vi "Host3.vi"() -> ()   [LabVIEW 2025]
uses:
  <vilib>/numeric/Random Number (Range) U64.vi
  <vilib>/Analysis/baseanly.llb/Real Dot Product.vi
  <vilib>/Analysis/baseanly.llb/Real A x B.vi
  <vilib>/numeric/sub_Random U32.vi
  <vilib>/Analysis/Matrix/Numeric/Conversions/Matrix To Array - RM.vi
  <vilib>/FPGAPlugInAG/cRIO-9033/niLvFpga_Open_cRIO-9033.vi
  <vilib>/rvi/interface/common/dynamic/niFpgaDynamicAddResources.vi
  <vilib>/FPGAPlugInAG/Dynamic/niLvFpga_Reset_Dynamic.vi
  <vilib>/Utility/error.llb/Error Cluster From Error Code.vi
  <vilib>/rvi/errors/niLvFpgaAdjustHostInterfaceError.vi
  <vilib>/FPGAPlugInAG/Dynamic/niLvFpga_Run_Dynamic.vi
  <vilib>/FPGAPlugInAG/Dynamic/niLvFpga_Close_Dynamic.vi
  <vilib>/rvi/interface/nirviOpenFPGA/nirviOpenFPGA.xnode
  FPGA Bitfiles/dotplot9033_FPGATarget_Target2_D+o9JZmHLrs.lvbitx
  Target2.vi
  <vilib>/rvi/interface/nirviMethod/nirviMethod.xnode
  <vilib>/rvi/interface/nirviReadWriteControl/nirviReadWriteControl.xnode
  <vilib>/rvi/interface/nirviCloseFPGA/nirviCloseFPGA.xnode
  <vilib>/rvi/errors/niLvFpgaMergeErrorWithErrorCode.vi
  <vilib>/Analysis/NI_AALBase.lvlib
  <vilib>/Analysis/Matrix/NI_Matrix.lvlib
  <vilib>/FPGAPlugInAG/Dynamic/niLvFpga_WriteFifo_Dynamic.vi
  <vilib>/FPGAPlugInAG/Dynamic/niLvFpga_ReadFifo_Dynamic.vi
  NiFpgaLv.dll
  <vilib>/rvi/interface/Simulation/niFpgaSimulationCallBeginRW.vi
panel:
  out "FIFO D.2 Output":fxp<+/-,32,16>[](array[numeric])
  out "Elements Remaining 4":u32
  out "FIFO C.2 Output":fxp<+/-,32,16>[](array[numeric])
  out "Elements Remaining 3":u32
  out "FIFO D Output":fxp<+/-,32,16>[](array[numeric])
  out "Elements Remaining 2":u32
  out "Array 1.2":fxp<+/-,32,16>[](array[numeric])
  out "Array 2.1":fxp<+/-,32,16>[](array[numeric])
  out "Array 2":fxp<+/-,32,16>[](array[numeric])
  out "Array 1":fxp<+/-,32,16>[](array[numeric])
  out "element 4":fxp<+/-,32,16>
  out "element 3":fxp<+/-,32,16>
  out "element 2":fxp<+/-,32,16>
  out "element":fxp<+/-,32,16>
  out "interleaved array 2":fxp<+/-,32,16>[](array[numeric])
  out "interleaved array":fxp<+/-,32,16>[](array[numeric])
  out "Case Number":i16
  out "Numeric":i32
  out "appended array 2":fxp<+/-,32,16>[](array[numeric])
  out "appended array":fxp<+/-,32,16>[](array[numeric])
  out "cr":fxp<+/-,32,16>[](array[numeric])
  out "Elements Remaining":u32
  out "FIFO C Output":fxp<+/-,32,16>[](array[numeric])
  out "FIFO A Input":fxp<+/-,32,16>[](array[numeric])
  out "FIFO B Input":fxp<+/-,32,16>[](array[numeric])
  out "X * Y":fxp<+/-,64,32>
  out "elements in B":i32
  out "elements in A":i32
  out "sum of error":dbl
  out "C - FPGA code":fxp<+/-,32,16>[][](array[numeric])
  out "elements in C":i32
  out "C - Real":dbl[][](array[numeric])
  out "B":fxp<+/-,32,16>[][](array[numeric])
  out "A":fxp<+/-,32,16>[][](array[numeric])
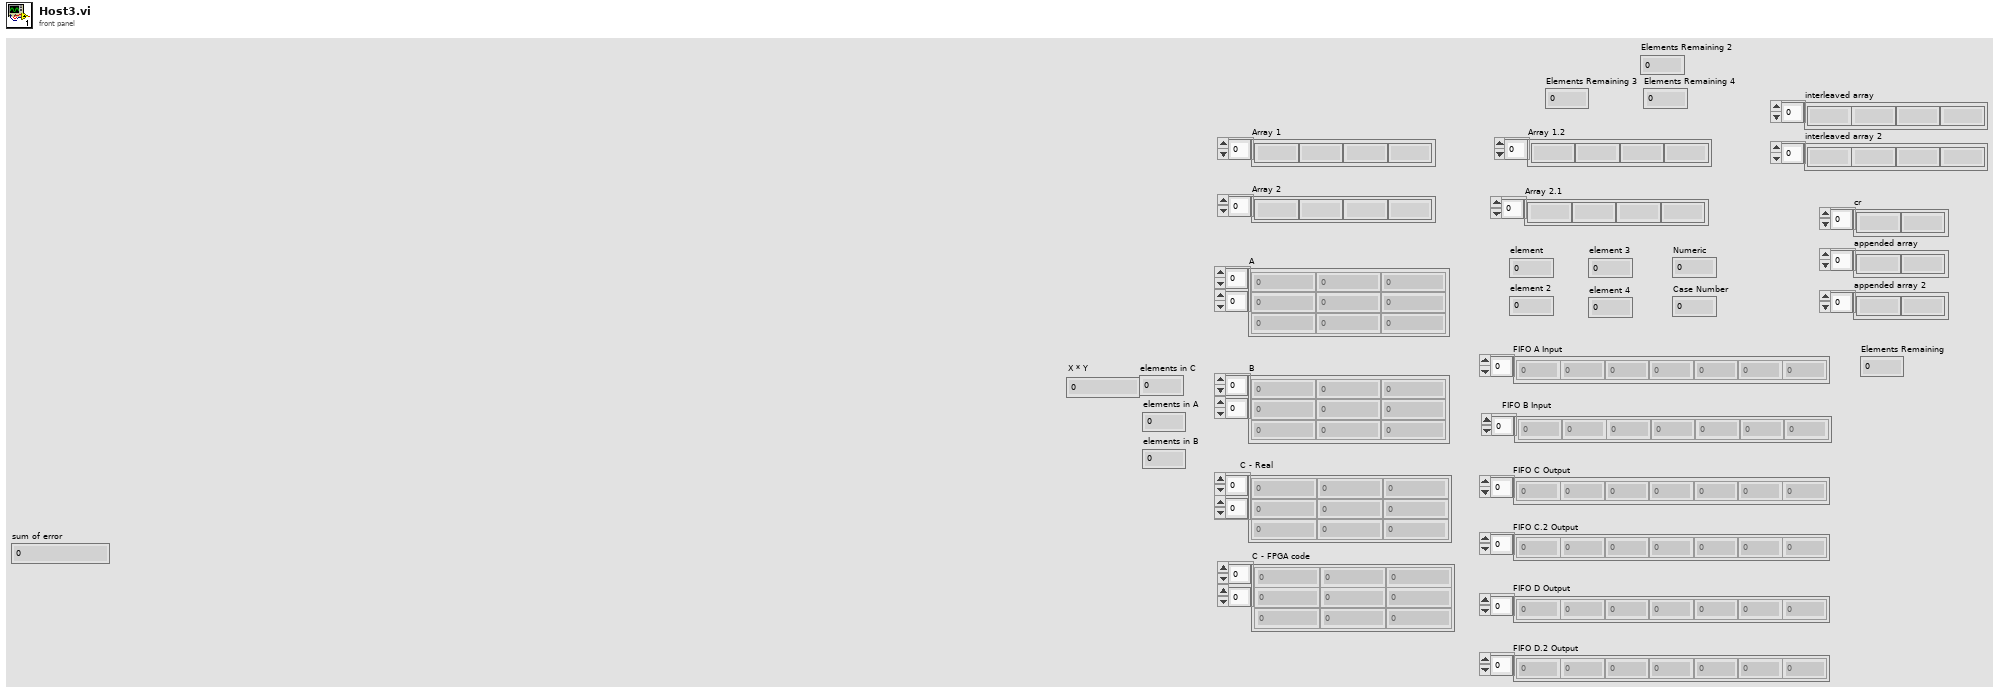
[diagram p1: front panel]
types:
  T1 = typedef "NI_Matrix.lvlib/RealMatrix.ctl" = dbl[][]
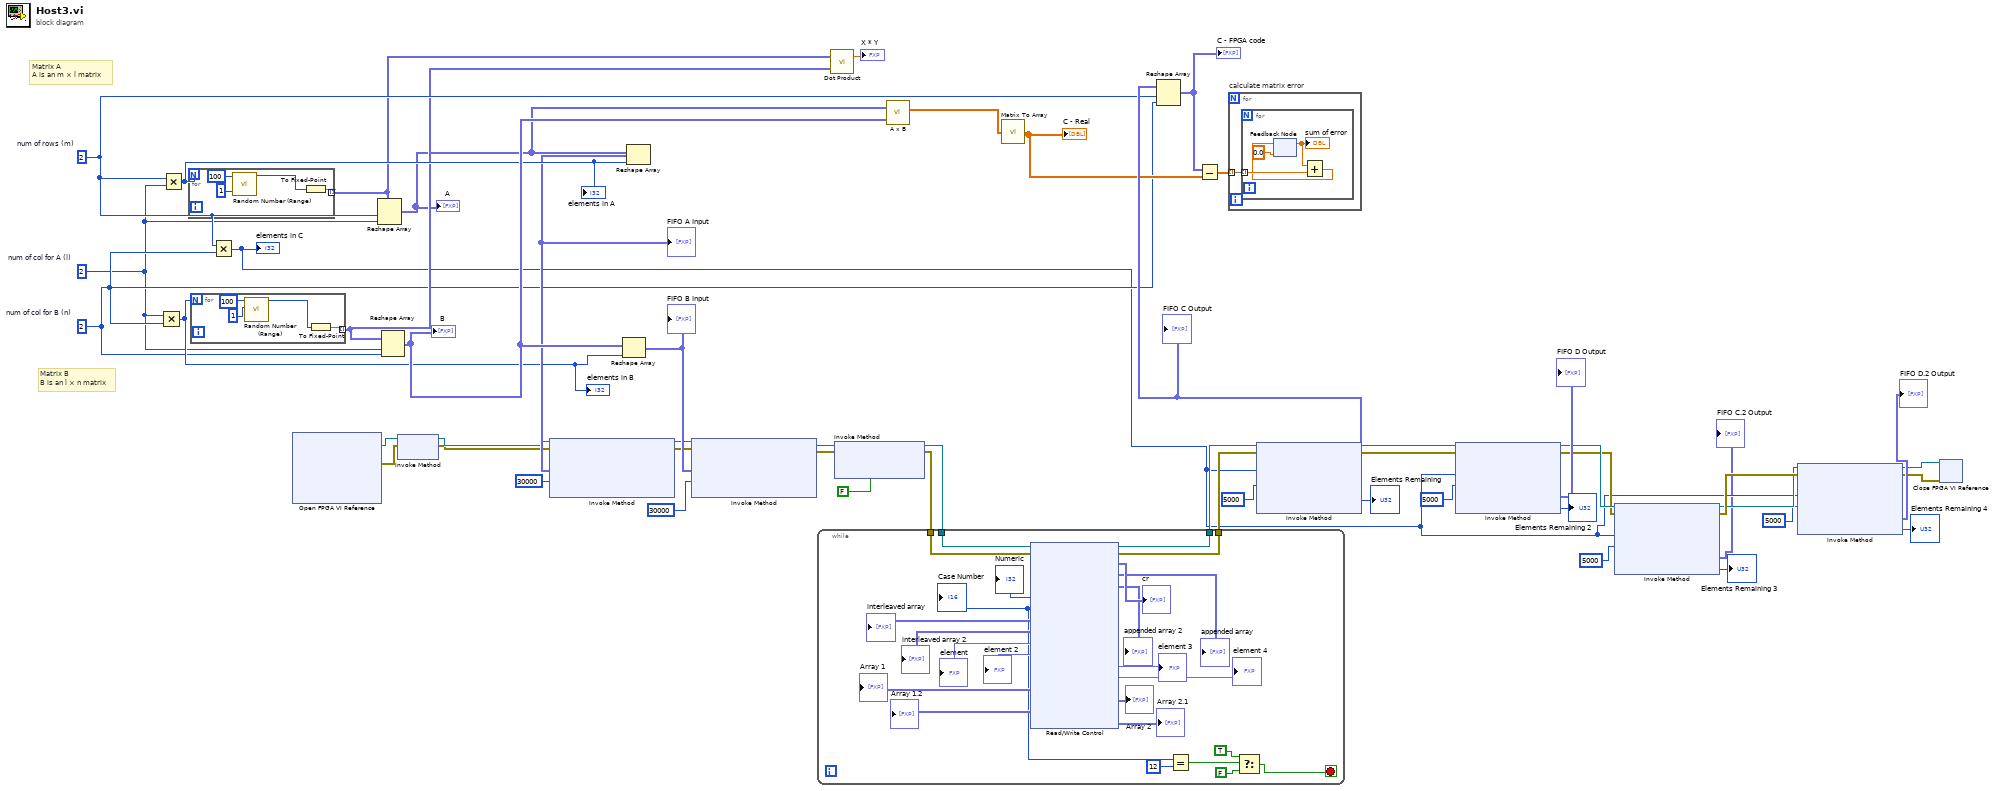
[diagram p0: block diagram]
diagram:
  w38 = 2  # num of col for B (n)
  w37 = 2  # num of col for A (l)
  w45 = 2  # num of rows (m)
  # "Matrix B\nB is an l × n matrix"
  # "Matrix A\nA is an m × l matrix"
  n1 = Multiply(x=w37, y=w38) -> (x*y=w43:i32)
  "elements in B" <- w43
  n2 = Multiply(x=w45, y=w37) -> (x*y=w50:i32)
  "elements in A" <- w50
  n3 = for {
    N: w50 -> [_]
    tunnel: [w56] -> w42 mode=indexing
    n4 = call-poly <vilib>:"Random Number (Range).vi"("lower bound (0)"=u64 1, "upper bound (100)"=u64 100) -> ("number"=w55:u64)  [unwired: 9 in]
    n5 = To Fixed-Point(number=w55) -> (fixed-point=w56:fxp<+,64,64>)  [unwired: 1 in]
  }
  n6 = for {
    N: w43 -> [_]
    tunnel: [w60] -> w41 mode=indexing
    n7 = call-poly <vilib>:"Random Number (Range).vi"("lower bound (0)"=u64 1, "upper bound (100)"=u64 100) -> ("number"=w57:u64)  [unwired: 9 in]
    n8 = To Fixed-Point(number=w57) -> (fixed-point=w60:fxp<+,64,64>)  [unwired: 1 in]
  }
  n9 = Multiply(x=w45, y=w38) -> (x*y=w7:i32)
  "elements in C" <- w7
  n10 = xnode "Open FPGA VI Reference"() -> ("FPGA VI Reference Out"=w35:refnum<k20>, "error out"=w32:errorcluster)  [unwired: 2 in]
  n11 = Reshape Array(w42, w45, w37) -> (w39:fxp<+,64,64>[][])
  "A" <- w39
  n12 = Reshape Array(w41, w37, w38) -> (w52:fxp<+,64,64>[][])
  "B" <- w52
  n13 = xnode "Invoke Method"("FPGA VI Reference In"=w35, "error in"=w32) -> ("FPGA VI Reference Out"=w34:refnum<k20>, "error out"=w33:errorcluster)
  n14 = Reshape Array(w52, w43) -> (w36:fxp<+,64,64>[])
  "FIFO B Input" <- w36
  n15 = Reshape Array(w39, w50) -> (w49:fxp<+,64,64>[])
  "FIFO A Input" <- w49
  n16 = xnode "Invoke Method"("FPGA VI Reference In"=w34, "error in"=w33, "Data"=w49, "Timeout (ms)"=30000) -> ("FPGA VI Reference Out"=w27:refnum<k20>, "error out"=w26:errorcluster)  [unwired: 1 out]
  n17 = xnode "Invoke Method"("FPGA VI Reference In"=w27, "error in"=w26, "Data"=w36, "Timeout (ms)"=30000) -> ("FPGA VI Reference Out"=w30:refnum<k20>, "error out"=w29:errorcluster)  [unwired: 1 out]
  n18 = call-poly <vilib>:"Dot Product.vi"("Y Vector"=w41, "X Vector"=w42) -> ("X * Y"=→"X * Y":dbl)  [unwired: 1 out]
  n19 = xnode "Invoke Method"("FPGA VI Reference In"=w30, "error in"=w29, "Wait Until Done (F)"=FALSE) -> ("FPGA VI Reference Out"=w22:refnum<k20>, "error out"=w21:errorcluster)
  n20 = while {
    tunnel: w22 -> [w70]
    tunnel: w21 -> [w69]
    tunnel: [w68] -> w20
    tunnel: [w67] -> w19
    stop <- w64 stop-if-true
    n21 = xnode "Read/Write Control"("FPGA VI Reference In"=w70, "error in"=w69) -> ("FPGA VI Reference Out"=w67:refnum<k20>, "error out"=w68:errorcluster, "cr"=→"cr":fxp<+/-,32,16>[], "appended array"=→"appended array":fxp<+/-,32,16>[], "appended array 2"=→"appended array 2":fxp<+/-,32,16>[], "Numeric"=→"Numeric":i32, "Case Number"=w66:i16, "interleaved array"=→"interleaved array":fxp<+/-,32,16>[], "interleaved array 2"=→"interleaved array 2":fxp<+/-,32,16>[], "element"=→"element":fxp<+/-,32,16>, "element 2"=→"element 2":fxp<+/-,32,16>, "element 3"=→"element 3":fxp<+/-,32,16>, "element 4"=→"element 4":fxp<+/-,32,16>, "Array 1"=→"Array 1":fxp<+/-,32,16>[], "Array 2"=→"Array 2":fxp<+/-,32,16>[], "Array 1.2"=→"Array 1.2":fxp<+/-,32,16>[], "Array 2.1"=→"Array 2.1":fxp<+/-,32,16>[])
    "Case Number" <- w66
    n22 = Equal?(x=w66, y=i16 12) -> (x = y?=w63:bool)
    n23 = Select(t=TRUE, s=w63, f=FALSE) -> (s? t:f=w64:bool)
  }
  n24 = call-poly <vilib>:"A x B.vi"("B"=w52, "A"=w39) -> ("A x B"=w51:T1)  [unwired: 1 out]
  n25 = call-poly <vilib>:"Matrix To Array.vi"("Real Matrix"=w51) -> ("Real 2D Array"=w44:dbl[][])
  "C - Real" <- w44
  n26 = xnode "Invoke Method"("FPGA VI Reference In"=w19, "error in"=w20, "Number of Elements"=w7, "Timeout (ms)"=5000) -> ("FPGA VI Reference Out"=w18:refnum<k20>, "error out"=w17:errorcluster, "Data"=w46:fxp<+/-,32,16>[], "Elements Remaining"=→"Elements Remaining":u32)
  "FIFO C Output" <- w46
  n27 = Reshape Array(w46, w45, w38) -> (w48:fxp<+/-,32,16>[][])
  "C - FPGA code" <- w48
  n28 = Subtract(x=w48, y=w44) -> (x-y=w47:dbl[][])
  n29 = for "calculate matrix error" {
    tunnel: w47 -> [w85] mode=indexing
    n30 = for {
      tunnel: w85 -> [w89] mode=indexing
      n31 = feedback #1(0.0) -> (w87:dbl)
      "sum of error" <- w87
      n32 = Add(x=w87, y=w89) -> (x+y=w88:dbl)
      n33 = feedback-in #1(w88) -> ()
    }
  }
  n34 = xnode "Invoke Method"("FPGA VI Reference In"=w18, "error in"=w17, "Number of Elements"=w7, "Timeout (ms)"=5000) -> ("FPGA VI Reference Out"=w13:refnum<k20>, "error out"=w12:errorcluster, "Data"=→"FIFO D Output":fxp<+/-,32,16>[], "Elements Remaining"=→"Elements Remaining 2":u32)
  n35 = xnode "Invoke Method"("FPGA VI Reference In"=w13, "error in"=w12, "Number of Elements"=w7, "Timeout (ms)"=5000) -> ("FPGA VI Reference Out"=w10:refnum<k20>, "error out"=w11:errorcluster, "Data"=→"FIFO C.2 Output":fxp<+/-,32,16>[], "Elements Remaining"=→"Elements Remaining 3":u32)
  n36 = xnode "Invoke Method"("FPGA VI Reference In"=w10, "error in"=w11, "Number of Elements"=w7, "Timeout (ms)"=5000) -> ("FPGA VI Reference Out"=w2:refnum<k20>, "error out"=w1:errorcluster, "Data"=→"FIFO D.2 Output":fxp<+/-,32,16>[], "Elements Remaining"=→"Elements Remaining 4":u32)
  n37 = xnode "Close FPGA VI Reference"("FPGA VI Reference In"=w2, "error in"=w1) -> ()  [unwired: 1 out]
